vi "CloseConection.vi"(8 "error in (no error)":errorcluster, 11 "NXP LPCXpresso54608 in":refnum<class "NXP LPCXpresso54608.lvclass">) -> (0 "error out":errorcluster, 3 "NXP LPCXpresso54608 out":refnum<class "NXP LPCXpresso54608.lvclass">)   [LabVIEW 2020, in "NXP LPCXpresso54608.lvclass"]
doc: "Close Conection from serial port."
uses:
  NXP LPCXpresso54608.lvclass
  NXP LPCXpresso54608.lvclass/NXP LPCXpresso54608.ctl
  Read Serial Port.vi
  Write Serial Port.vi
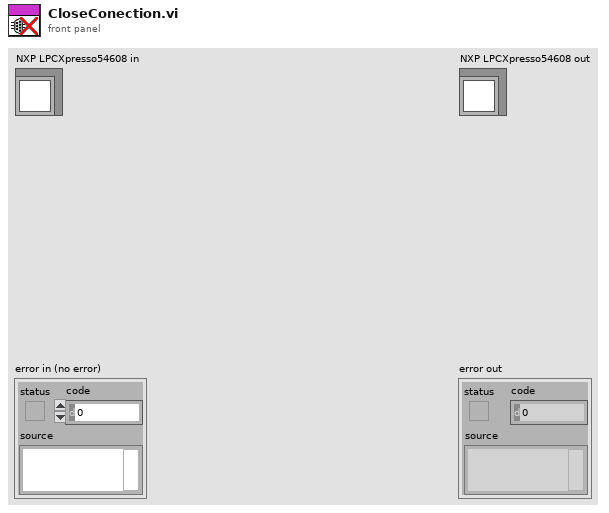
[diagram p1: front panel]
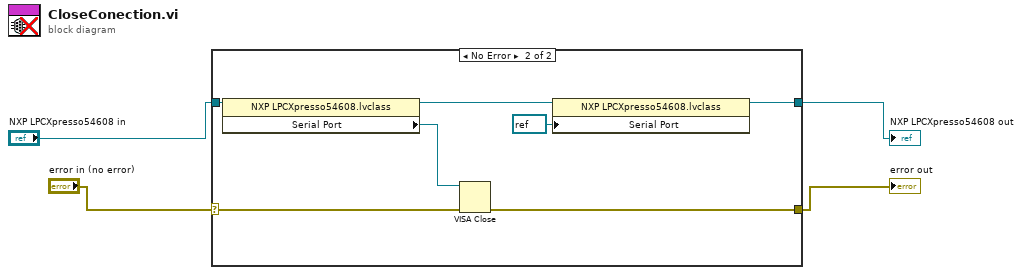
[diagram p0: block diagram]
diagram:
  n1 = case shown="No Error" "error in (no error)" {
    selector: "error in (no error)" -> [w5 w12]
    tunnel: "NXP LPCXpresso54608 in" -> [w6 w13]
    tunnel: [w6 w8] -> w1
    tunnel: [w5 w10] -> w2
    frame Error {
    }
    frame No Error {
      n2 = property class="NXP LPCXpresso54608.lvclass"(reference=w13) -> (reference out=w11:refnum<class "NXP LPCXpresso54608.lvclass">, "Serial Port"=w9:refnum<visa-resource-name>)  [unwired: 1 in, 1 out]
      n3 = VISA Close(VISA resource name=w9, error in (no error)=w12) -> (error out=w10:errorcluster)
      n4 = property class="NXP LPCXpresso54608.lvclass"(reference=w11, "Serial Port"=refnum<visa-resource-name> refnum) -> (reference out=w8:refnum<class "NXP LPCXpresso54608.lvclass">)  [unwired: 1 in, 1 out]
    }
  }
  "error out" <- w2
  "NXP LPCXpresso54608 out" <- w1
